vi "GUI_Bella_BTL.vi"() -> ()   [LabVIEW 2013]
uses:
  <vilib>/vision/Image Controls.llb/IMAQ Image.ctl
  shared programs/GUI_Template/GUI_master/tcp new data cluster.ctl
  shared programs/GUI_Template/GUI_master/tcp_new_data_event.ctl
  Device Driver/LEPS Interface/Filter_typdef.ctl
panel:
  out "x >= y?":bool
  in  "stepsize::6":dbl=0.001 caption="Step Size" min=0.0 max=1.0 format="%.3f"
  in  "stepsize::7":dbl=0.001 caption="Step Size" min=0.0 max=1.0 format="%.3f"
  in  "stepsize::8":dbl=0.001 caption="Step Size" min=0.0 max=1.0 format="%.3f"
  in  "size1":dbl=20.0 caption="Size" min=0.0 max=0.0
  in  "Target.X::1":dbl=0.001 caption="X" min=0.0 max=2000.0
  in  "Target.Y::1":dbl=0.001 caption="Y" min=0.0 max=2000.0
  in  "centroidx::1":dbl=0.001 caption="X" min=0.0 max=0.0
  in  "centroidy::1":dbl=0.001 caption="Y" min=0.0 max=0.0
  in  "trigger::1":bool caption="Blank Button"
  in  "exposure::1":dbl=0.001 caption="Exposure" min=3.8e-05 max=1.0 format="%_4p"
  in  "filter.var 1::9":T1=enum."OD1" caption="Filter Wheel"
  in  "relativeMove.Axis 1neg::7":bool
  in  "relativeMove.Axis 1pos::7":bool
  in  "relativeMove.Axis 2pos::7":bool
  in  "relativeMove.Axis 2neg::7":bool
  in  "size3":dbl=20.0 caption="Size" min=0.0 max=0.0
  in  "Target.X::3":dbl=0.001 caption="X" min=0.0 max=2000.0
  in  "Target.Y::3":dbl=0.001 caption="Y" min=0.0 max=2000.0
  in  "centroidx::3":dbl=0.001 caption="X" min=0.0 max=0.0
  in  "centroidy::3":dbl=0.001 caption="Y" min=0.0 max=0.0
  in  "trigger::3":bool caption="Blank Button"
  in  "exposure::3":dbl=0.001 caption="Exposure" min=3.8e-05 max=1.0 format="%_4p"
  in  "filter.var 4::9":T1=enum."OD1" caption="Filter Wheel"
  in  "relativeMove.Axis 2neg::6":bool
  in  "relativeMove.Axis 2pos::6":bool
  in  "relativeMove.Axis 3pos::6":bool
  in  "relativeMove.Axis 3neg::6":bool
  in  "size4":dbl=20.0 caption="Size" min=0.0 max=0.0
  in  "Target.X::4":dbl=0.001 caption="X" min=0.0 max=2000.0
  in  "Target.Y::4":dbl=0.001 caption="Y" min=0.0 max=2000.0
  in  "centroidx::4":dbl=0.001 caption="X" min=0.0 max=0.0
  in  "centroidy::4":dbl=0.001 caption="Y" min=0.0 max=0.0
  in  "trigger::4":bool caption="Blank Button"
  in  "exposure::4":dbl=0.001 caption="Exposure" min=3.8e-05 max=1.0 format="%_4p"
  in  "relativeMove.Axis 1neg::8":bool
  in  "relativeMove.Axis 1pos::8":bool
  in  "relativeMove.Axis 2pos::8":bool
  in  "relativeMove.Axis 2neg::8":bool
  in  "size5":dbl=25.0 caption="Size" min=0.0 max=0.0
  in  "Target.X::5":dbl=0.001 caption="X" min=0.0 max=2000.0
  in  "Target.Y::5":dbl=0.001 caption="Y" min=0.0 max=2000.0
  in  "centroidx::5":dbl=0.001 caption="X" min=0.0 max=0.0
  in  "centroidy::5":dbl=0.001 caption="Y" min=0.0 max=0.0
  in  "trigger::5":bool caption="Blank Button"
  in  "exposure::5":dbl=0.001 caption="Exposure" min=3.8e-05 max=1.0 format="%_4p"
  in  "filter.var 2::9":T1=enum."OD1" caption="Filter Wheel"
  in  "relativeMove.Axis 1pos::6":bool
  in  "relativeMove.Axis 1neg::6":bool
  in  "relativeMove.Axis 3pos::7":bool
  in  "relativeMove.Axis 3neg::7":bool
  out "image::5":T2(plugin-control) caption="M1 Cam"
  out "image::4":T2(plugin-control) caption="M1 Cam"
  out "image::3":T2(plugin-control) caption="M1 Cam"
  in  "size2":dbl=20.0 caption="Size" min=0.0 max=0.0
  out "image::2":T2(plugin-control) caption="M1 Cam"
  out "image::1":T2(plugin-control) caption="M1 Cam"
  in  "GUIdevice 9":string="71146 LEPS Interface"
  out "tcp data event":T3
  in  "Target.X::2":dbl=0.001 caption="X" min=0.0 max=2000.0
  in  "Target.Y::2":dbl=0.001 caption="Y" min=0.0 max=2000.0
  in  "GUIdevice 8":string="BELLA_ESP_M1"
  in  "GUIdevice 7":string="BellaESP"
  in  "GUIdevice 6":string="BELLA_ESP_2"
  in  "centroidx::2":dbl=0.001 caption="X" min=0.0 max=0.0
  in  "centroidy::2":dbl=0.001 caption="Y" min=0.0 max=0.0
  in  "trigger::2":bool caption="Blank Button"
  in  "GUIdevice 5":string="M2Cam"
  out "Display5":T2(plugin-control) caption="M1 Cam"
  in  "GUIdevice 4":string="Bella_LP_Mode"
  out "Display4":T2(plugin-control) caption="M1 Cam"
  in  "GUIdevice 3":string="M4Cam"
  out "Display3":T2(plugin-control) caption="M1 Cam"
  in  "exposure::2":dbl=0.001 caption="Exposure" min=3.8e-05 max=1.0 format="%_4p"
  in  "GUIdevice 2":string="M5Cam"
  in  "filter.var 5::9":T1=enum."OD1" caption="Filter Wheel"
  out "Display2":T2(plugin-control) caption="M1 Cam"
  in  "stop":bool
  in  "GUIdevice 1":string="M1Cam"
  out "error IO 2":errorcluster
  out "Display1":T2(plugin-control) caption="M1 Cam"
  # "Target"
  # "Centroid"
  # "Target"
  # "Centroid"
  # "Target"
  # "Centroid"
  # "Target"
  # "Centroid"
  # "M5 X-Axis, LP Mode CAMS"
  # "M5 Y-Axis, M4 CAMS"
  # "Target"
  # "Centroid"
  # "M2 CAM"
  # "M5 and LP Mode CAMS"
  # "M4 and M5 CAMS"
  # "M2 CAM"
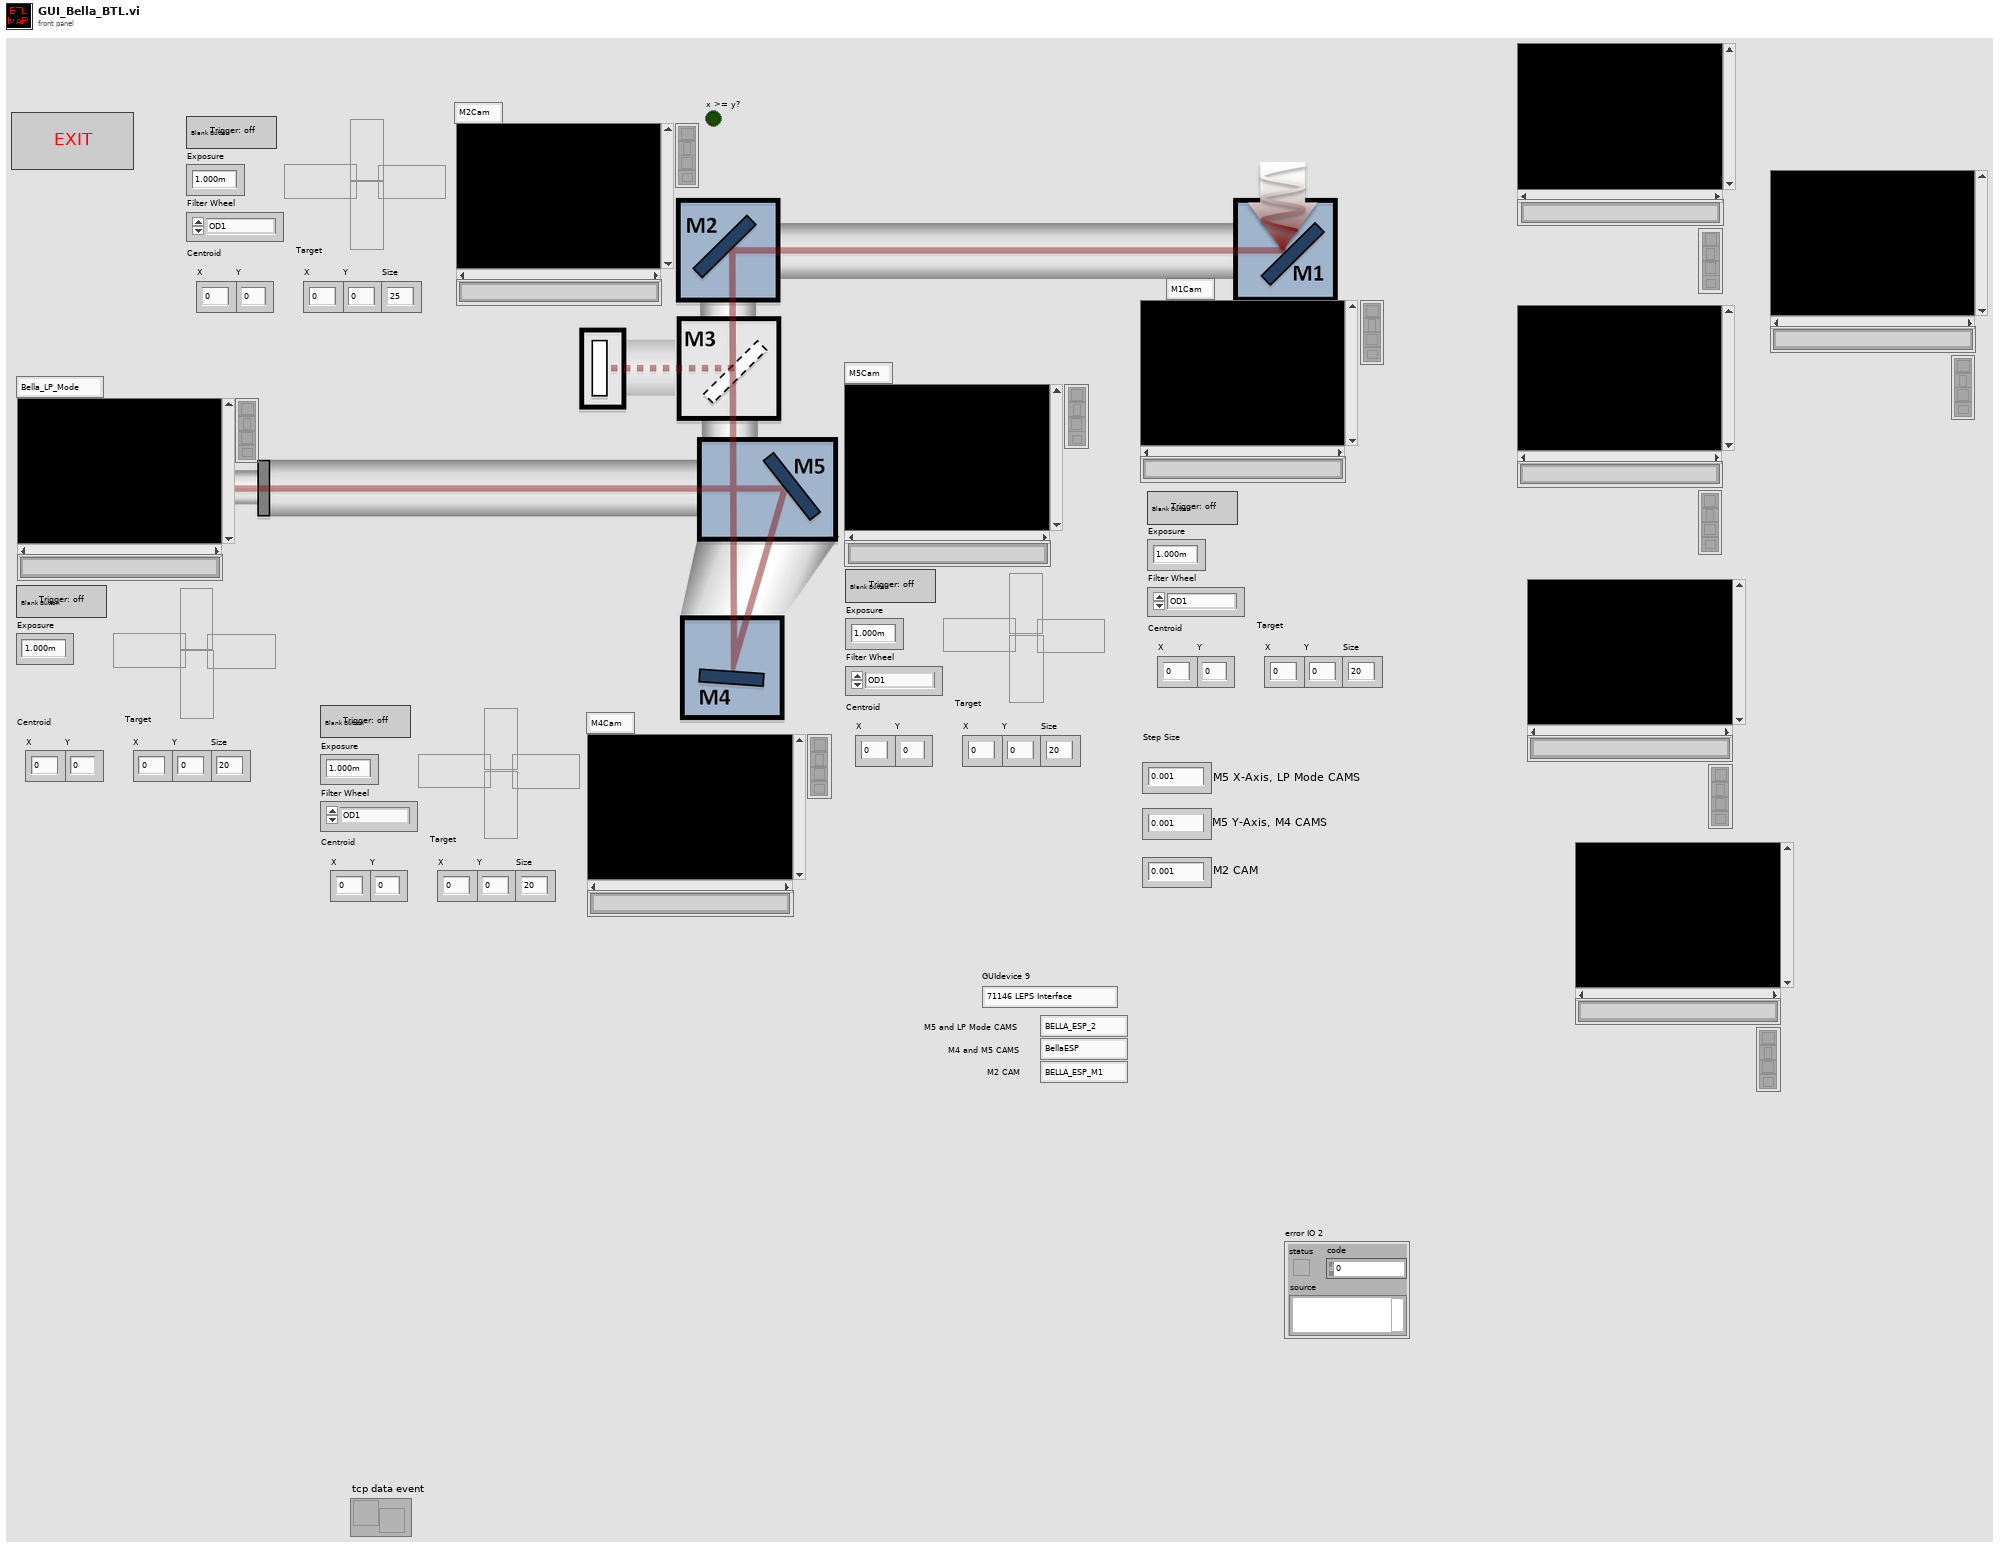
[diagram p1: front panel]
types:
  T1 = typedef "Filter_typdef.ctl" = enum16{"Moving/Unknown", "OD1", "OD2", "OD3", "OD4", "OD5", "Open(6)"}
  T2 = typedef "IMAQ Image.ctl" = refnum<image>
  T3 = typedef "tcp_new_data_event.ctl" = refnum<user-event>
  T4 = typedef "Image Type" = u32
  T5 = typedef "tcp new data cluster.ctl" = cluster{"EventEnum":enum16{"new data", "connection status update"}, "Device name":string}
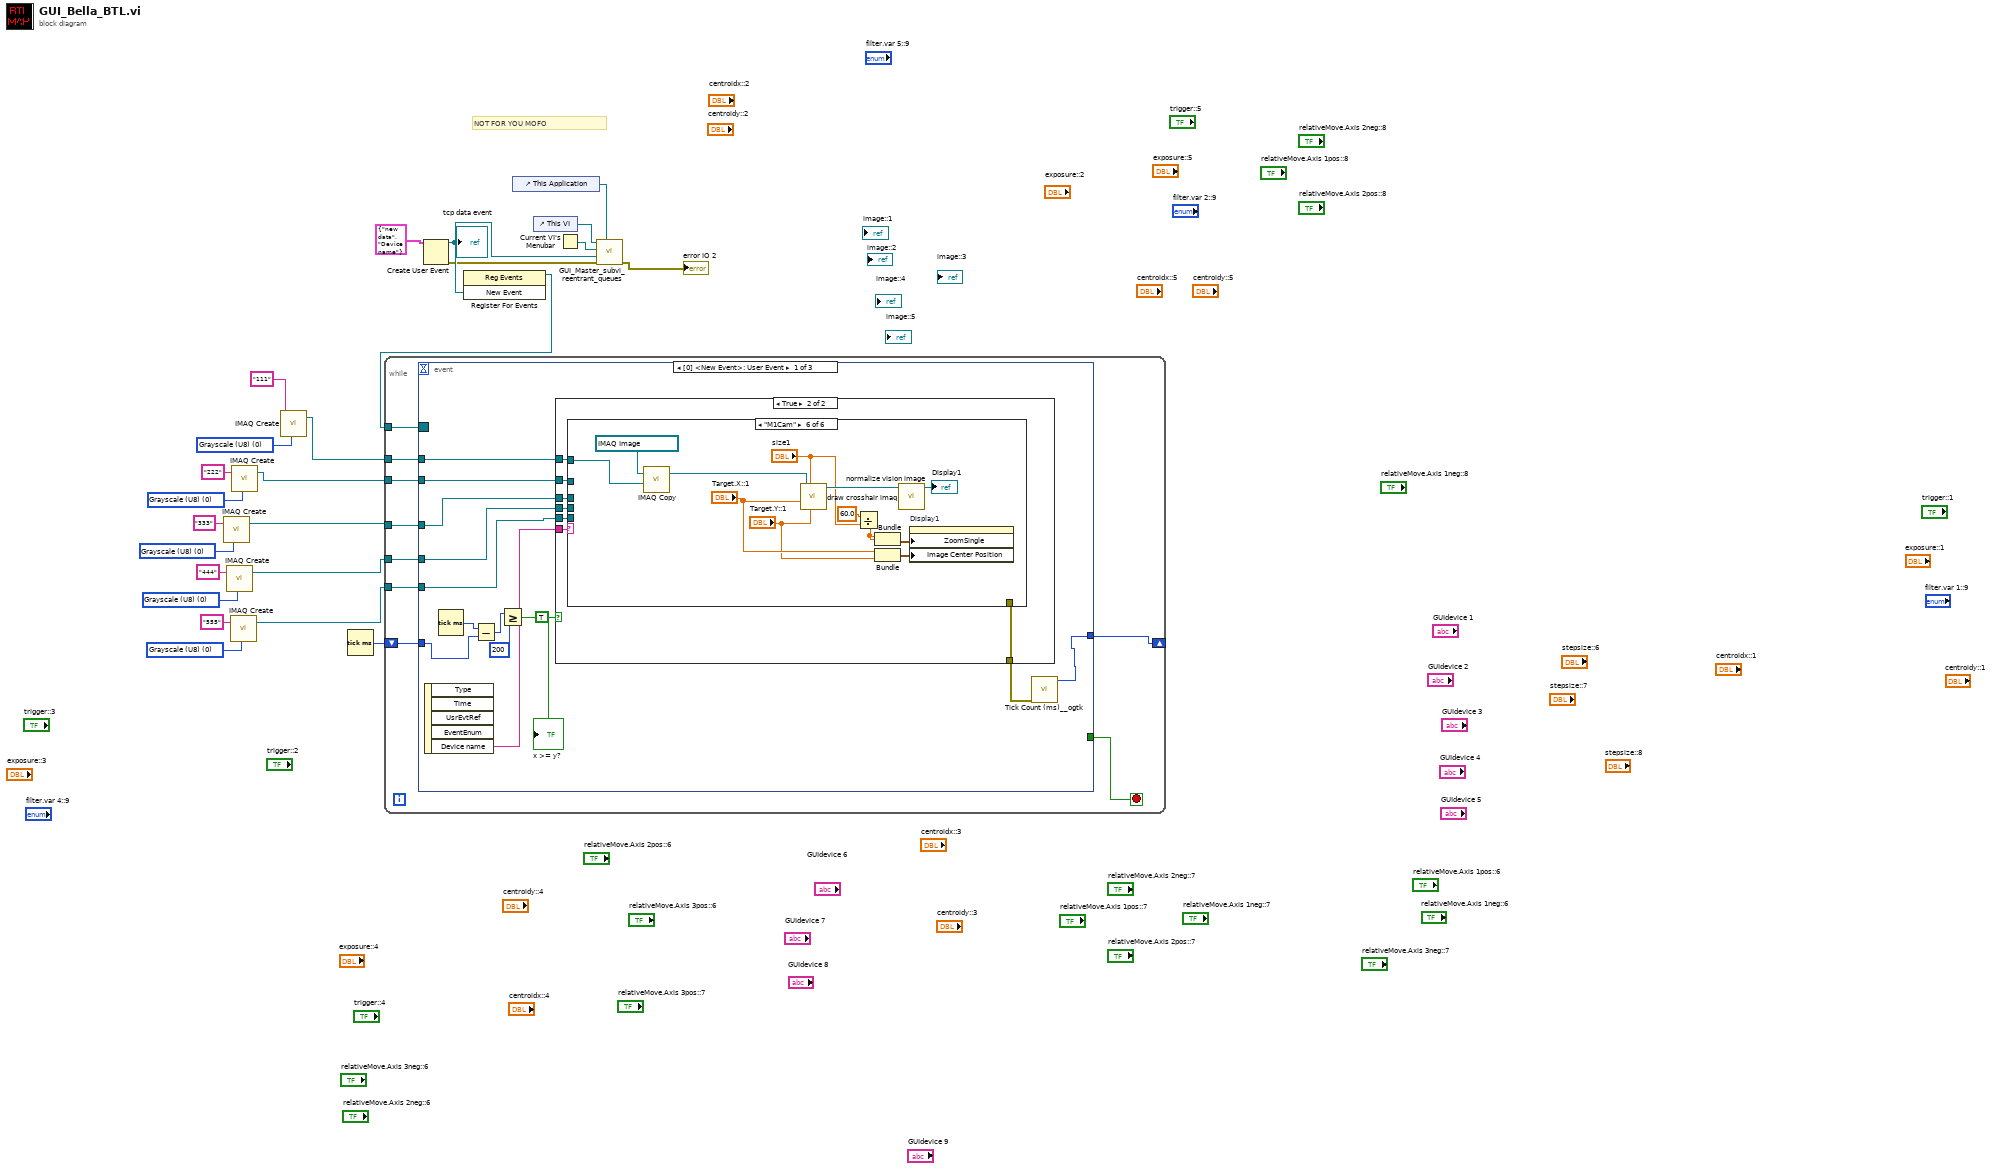
[diagram p0: block diagram]
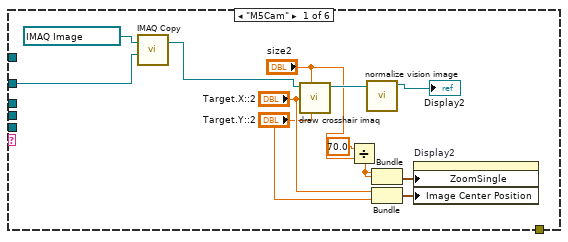
[diagram p3: hidden frame]
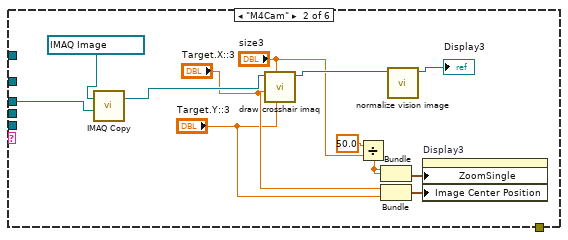
[diagram p4: hidden frame]
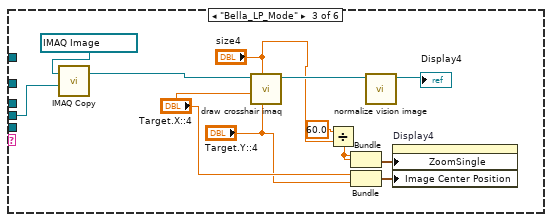
[diagram p5: hidden frame]
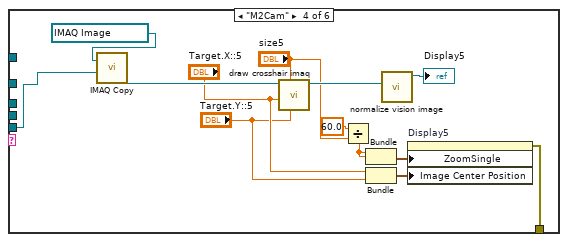
[diagram p6: hidden frame]
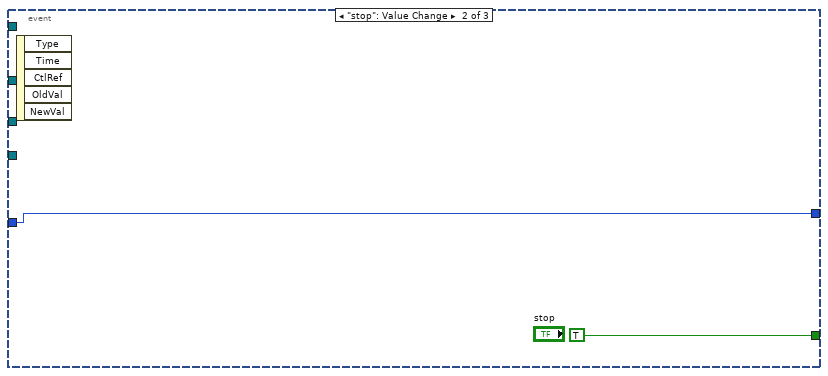
[diagram p8: hidden frame]
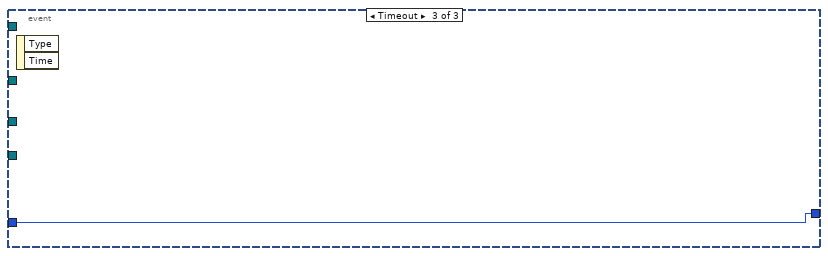
[diagram p9: hidden frame]
diagram:
  w3 = T4 0 items=["Grayscale (U8)", "Grayscale (I16)", "Grayscale (SGL)", "Complex (CSG)", "RGB (U32)", "HSL (U32)", "RGB (U64)", "Grayscale (U16)"] ("Image Type")
  w7 = T4 0 items=["Grayscale (U8)", "Grayscale (I16)", "Grayscale (SGL)", "Complex (CSG)", "RGB (U32)", "HSL (U32)", "RGB (U64)", "Grayscale (U16)"] ("Image Type")
  w9 = T4 0 items=["Grayscale (U8)", "Grayscale (I16)", "Grayscale (SGL)", "Complex (CSG)", "RGB (U32)", "HSL (U32)", "RGB (U64)", "Grayscale (U16)"] ("Image Type")
  w13 = T4 0 items=["Grayscale (U8)", "Grayscale (I16)", "Grayscale (SGL)", "Complex (CSG)", "RGB (U32)", "HSL (U32)", "RGB (U64)", "Grayscale (U16)"] ("Image Type")
  w14 = T4 0 items=["Grayscale (U8)", "Grayscale (I16)", "Grayscale (SGL)", "Complex (CSG)", "RGB (U32)", "HSL (U32)", "RGB (U64)", "Grayscale (U16)"] ("Image Type")
  # "NOT FOR YOU MOFO"
  n1 = call "IMAQ Create"("Image Name"="333", "Image Type"=w9) -> ("New Image"=w8:T2)  [unwired: 3 in, 1 out]
  n2 = call "IMAQ Create"("Image Name"="444", "Image Type"=w7) -> ("New Image"=w5:T2)  [unwired: 3 in, 1 out]
  n3 = call "IMAQ Create"("Image Name"="555", "Image Type"=w3) -> ("New Image"=w2:T2)  [unwired: 3 in, 1 out]
  n4 = call "IMAQ Create"("Image Name"="222", "Image Type"=w13) -> ("New Image"=w11:T2)  [unwired: 3 in, 1 out]
  n5 = call "IMAQ Create"("Image Name"="111", "Image Type"=w14) -> ("New Image"=w15:T2)  [unwired: 3 in, 1 out]
  n6 = Tick Count (ms)() -> (millisecond timer value=w1:u32)
  n7 = Create User Event(user event datatype=T5 {"EventEnum"=enum."new data", "Device name"="Device name"} ("New Event")) -> (user event=w23:refnum<user-event>, error out=w22:errorcluster)  [unwired: 1 in]
  "tcp data event" <- w23
  n8 = register-events(w23) -> (reference out=w18:refnum<event-registration>)  [unwired: 2 in, 1 out]
  n9 = while {
    tunnel: w18 -> [w32]
    tunnel: w15 -> [w31]
    tunnel: w11 -> [w30]
    tunnel: w8 -> [w29]
    tunnel: w5 -> [w28]
    tunnel: w2 -> [w27]
    shift-right: [w25] -> _
    shift-left: w1 -> [w26]
    stop <- w33 stop-if-true
    n10 = event shown="[0] <New Event>: User Event" {
      selector: w32 -> [_ _ _]
      dyn-events: _ -> [_ _ _]
      timeout: _ -> [_ _ _]
      tunnel: [_ TRUE ("stop") _] -> w33
      tunnel: w31 -> [w47 _ _]
      tunnel: w30 -> [w45 _ _]
      tunnel: w29 -> [w44 _ _]
      tunnel: w28 -> [w43 _ _]
      tunnel: w27 -> [w42 _ _]
      tunnel: w26 -> [w41 w116 w118]
      tunnel: [w37 w116 w118] -> w25
      event User Event {
        n11 = event-data() -> ("Device name"=w46:string)  [unwired: 1 in, 4 out]
        n12 = Tick Count (ms)() -> (millisecond timer value=w38:u32)
        n13 = Subtract(x=w38, y=w41) -> (x-y=w40:u32)
        n14 = Greater Or Equal?(x=w40, y=u32 200 ("x-y")) -> (x >= y?=→"x >= y?":bool)
        n15 = case shown="True" TRUE {
          tunnel: w47 -> [_ w54]
          tunnel: w46 -> [_ w53]
          tunnel: w45 -> [_ w52]
          tunnel: w44 -> [_ w51]
          tunnel: w43 -> [_ w50]
          tunnel: w42 -> [_ w49]
          tunnel: [_ w48] -> w36
          frame False {
          }
          frame True {
            n16 = case shown="\"M1Cam\"" w53 {
              tunnel: w54 -> [_ _ _ _ _ w112]
              tunnel: w52 -> [w65 _ _ _ _ _]
              tunnel: w51 -> [_ w77 _ _ _ _]
              tunnel: w50 -> [_ _ w87 _ _ _]
              tunnel: w49 -> [_ _ _ w102 _ _]
              tunnel: [_ _ _ w91 _ _] -> w48
              frame "M5Cam" {
                n17 = call "IMAQ Copy"("Image Dst"=w65, "Image Src"=T2 refnum ("New Image")) -> ("Image Dst Out"=w64:T2)  [unwired: 4 in, 1 out]
                n18 = call "draw crosshair imaq.vi"("Target.Y"="Target.Y::2", "size"="size2", "Target.X"="Target.X::2", "image in"=w64) -> ("image out"=w63:T2)  [unwired: 6 in, 1 out]
                n19 = Divide(x=70.0, y="size2") -> (x/y=w59:dbl)
                n20 = call "normalize vision image.vi"("Refnum in"=w63) -> ("Refnum out"=→"Display2":T2)  [unwired: 8 in, 2 out]
                n21 = Bundle(w59, w59) -> (w61:cluster{dbl, dbl})  [unwired: 1 in]
                n22 = Bundle("Target.X::2"="Target.X::2", "Target.Y::2"="Target.Y::2") -> (w58:cluster{"Target.X::2":dbl, "Target.Y::2":dbl})  [unwired: 1 in]
                n23 = property on="Display2" class="ImageControl"("ZoomSingle"=w61, "Image Center Position"=w58) -> ()  [unwired: 2 in, 2 out]
              }
              frame "M4Cam" {
                n24 = call "IMAQ Copy"("Image Dst"=w77, "Image Src"=T2 refnum ("New Image")) -> ("Image Dst Out"=w76:T2)  [unwired: 4 in, 1 out]
                n25 = call "draw crosshair imaq.vi"("Target.Y"="Target.Y::3", "size"="size3", "Target.X"="Target.X::3", "image in"=w76) -> ("image out"=w75:T2)  [unwired: 6 in, 1 out]
                n26 = Divide(x=50.0, y="size3") -> (x/y=w71:dbl)
                n27 = Bundle(w71, w71) -> (w73:cluster{dbl, dbl})  [unwired: 1 in]
                n28 = Bundle("Target.X::3"="Target.X::3", "Target.Y::3"="Target.Y::3") -> (w70:cluster{"Target.X::3":dbl, "Target.Y::3":dbl})  [unwired: 1 in]
                n29 = call "normalize vision image.vi"("Refnum in"=w75) -> ("Refnum out"=→"Display3":T2)  [unwired: 8 in, 2 out]
                n30 = property on="Display3" class="ImageControl"("ZoomSingle"=w73, "Image Center Position"=w70) -> ()  [unwired: 2 in, 2 out]
              }
              frame "Bella_LP_Mode" {
                n31 = call "IMAQ Copy"("Image Dst"=w87, "Image Src"=T2 refnum ("New Image")) -> ("Image Dst Out"=w86:T2)  [unwired: 4 in, 1 out]
                n32 = call "draw crosshair imaq.vi"("Target.Y"="Target.Y::4", "size"="size4", "Target.X"="Target.X::4", "image in"=w86) -> ("image out"=w90:T2)  [unwired: 6 in, 1 out]
                n33 = Divide(x=60.0, y="size4") -> (x/y=w83:dbl)
                n34 = Bundle(w83, w83) -> (w85:cluster{dbl, dbl})  [unwired: 1 in]
                n35 = Bundle("Target.X::4"="Target.X::4", "Target.Y::4"="Target.Y::4") -> (w82:cluster{"Target.X::4":dbl, "Target.Y::4":dbl})  [unwired: 1 in]
                n36 = call "normalize vision image.vi"("Refnum in"=w90) -> ("Refnum out"=→"Display4":T2)  [unwired: 8 in, 2 out]
                n37 = property on="Display4" class="ImageControl"("ZoomSingle"=w85, "Image Center Position"=w82) -> ()  [unwired: 2 in, 2 out]
              }
              frame "M2Cam" {
                n38 = call "IMAQ Copy"("Image Dst"=w102, "Image Src"=T2 refnum ("New Image")) -> ("Image Dst Out"=w103:T2)  [unwired: 4 in, 1 out]
                n39 = call "draw crosshair imaq.vi"("Target.Y"="Target.Y::5", "size"="size5", "Target.X"="Target.X::5", "image in"=w103) -> ("image out"=w100:T2)  [unwired: 6 in, 1 out]
                n40 = Divide(x=60.0, y="size5") -> (x/y=w96:dbl)
                n41 = Bundle(w96, w96) -> (w98:cluster{dbl, dbl})  [unwired: 1 in]
                n42 = Bundle("Target.X::5"="Target.X::5", "Target.Y::5"="Target.Y::5") -> (w95:cluster{"Target.X::5":dbl, "Target.Y::5":dbl})  [unwired: 1 in]
                n43 = call "normalize vision image.vi"("Refnum in"=w100) -> ("Refnum out"=→"Display5":T2)  [unwired: 8 in, 2 out]
                n44 = property on="Display5" class="ImageControl"("ZoomSingle"=w98, "Image Center Position"=w95) -> (error out=w91:errorcluster)  [unwired: 2 in, 1 out]
              }
              frame Default {
              }
              frame "M1Cam" {
                n45 = call "IMAQ Copy"("Image Dst"=w112, "Image Src"=T2 refnum ("New Image")) -> ("Image Dst Out"=w111:T2)  [unwired: 4 in, 1 out]
                n46 = call "draw crosshair imaq.vi"("Target.Y"="Target.Y::1", "size"="size1", "Target.X"="Target.X::1", "image in"=w111) -> ("image out"=w115:T2)  [unwired: 6 in, 1 out]
                n47 = Divide(x=60.0, y="size1") -> (x/y=w108:dbl)
                n48 = Bundle(w108, w108) -> (w110:cluster{dbl, dbl})  [unwired: 1 in]
                n49 = Bundle("Target.X::1"="Target.X::1", "Target.Y::1"="Target.Y::1") -> (w104:cluster{"Target.X::1":dbl, "Target.Y::1":dbl})  [unwired: 1 in]
                n50 = call "normalize vision image.vi"("Refnum in"=w115) -> ("Refnum out"=→"Display1":T2)  [unwired: 8 in, 2 out]
                n51 = property on="Display1" class="ImageControl"("ZoomSingle"=w110, "Image Center Position"=w104) -> ()  [unwired: 2 in, 2 out]
              }
            }
          }
        }
        n52 = call <userlib>:"Tick Count (ms)__ogtk.vi"("error in (no error)"=w36) -> ("millisecond timer value"=w37:u32)  [unwired: 9 in, 1 out]
      }
      event "stop": Value Change {
        n53 = event-data() -> ()  [unwired: 1 in, 5 out]
      }
      event Timeout {
        n54 = event-data() -> ()  [unwired: 1 in, 2 out]
      }
    }
  }
  n55 = control-ref of="This Application"() -> (w24:refnum<vi>)
  n56 = control-ref of="This VI"() -> (w19:refnum<vi>)
  n57 = Current VI's Menubar() -> (w20:refnum<k9>)
  n58 = call "GUI_Master_subvi_reentrant_queues.vi"("This Application"=w24, "error in (no error)"=w22, "tcp data event"=w23, "Caller menu reference"=w20, "Caller VI ref"=w19) -> ("error out"=→"error IO 2":errorcluster)  [unwired: 6 in]
